vi "Extract_MCU_name_from_array.vi"(3 "Input Array":dbl[](array[numeric])) -> (0 "In Range?":bool, 1 "MCU Name":string)   [LabVIEW 2016]
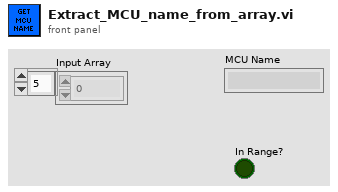
[diagram p1: front panel]
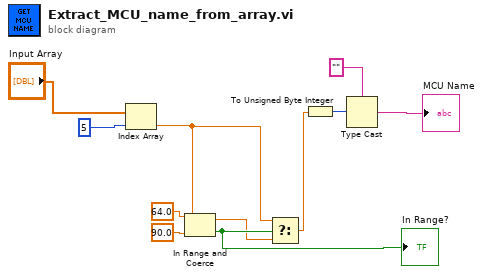
[diagram p0: block diagram]
diagram:
  n1 = Index Array(array="Input Array", index=5 ("index 4")) -> (element=w1:dbl)
  n2 = In Range and Coerce(upper limit=64.0, x=w1, lower limit=90.0) -> (coerced(x)=w2:dbl, In Range?=w4:bool)
  "In Range?" <- w4
  n3 = Select(t=w1, s=w4, f=w2) -> (s? t:f=w3:dbl)
  n4 = To Unsigned Byte Integer(number=w3) -> (unsigned 8bit integer=w10:u8)
  n5 = Type Cast(type="", x=w10) -> (*(type *) &x=→"MCU Name":string)
